vi "Performance Test.vi"() -> ()   [LabVIEW 2017]
uses:
  <vilib>/Simulation/Implementation/Shared/SIMSCR Execution Mode.ctl
  <vilib>/Simulation/Scripting/Companion Diagram/SimConfigNode/_simSolvers.ctl
  <vilib>/Simulation/Scripting/Companion Diagram/SimConfigNode/SimParams.ctl
  <vilib>/Simulation/Scripting/Companion Diagram/SimConfigNode/SimDog.xnode
  <vilib>/Simulation/Implementation/XNodeFramework/SimXNode/SimX.xnode
  FPGA_Read_Write.vi
  Manipulator/Inv Kin.vi
  Manipulator/Fwd Kin.vi
  Extras/type convert.vi
  <extravilib>/ChannelInstances/Tag-a[.](dbl).lvlib
  <extravilib>/ChannelInstances/Tag-bool.lvlib
  <vilib>/Platform/TimedLoop/XDataNode/wakeup.ctl
  <vilib>/Platform/TimedLoop/XDataNode/XDNodeRunTimeDep.lvlib
  <vilib>/Platform/TimedLoop/XDataNode/nitl_modes.ctl
  <vilib>/Platform/TimedLoop/XDataNode/timing_clust.ctl
  <vilib>/Platform/TimedLoop/XDataNode/XDataNode.xnode
  <extravilib>/ChannelInstances/Tag-c(bool,i32,str).lvlib
  <extravilib>/ChannelInstances/Tag-a[.](c(dbl,dbl)).lvlib
  Extras/NaN Check.vi
  <vilib>/rvi/interface/nirviReadWriteControl/nirviReadWriteControl.xnode
  <extravilib>/ChannelInstances/Tag-dbl.lvlib
  <vilib>/Analysis/baseanly.llb/Dot Product.vi
  <vilib>/Analysis/NI_AALBase.lvlib
  <vilib>/Analysis/baseanly.llb/Real Dot Product.vi
  <extravilib>/ChannelInstances/Tag-a[.](i32).lvlib
  Calibration/c PID.vi
  NiFpgaLv.dll
  <vilib>/Utility/error.llb/Error Cluster From Error Code.vi
  <vilib>/rvi/interface/Simulation/niFpgaSimulationCallBeginRW.vi
  <vilib>/rvi/errors/niLvFpgaAdjustHostInterfaceError.vi
  <vilib>/Simulation/Utility/Implementation/SIM Time.vi
  <vilib>/Simulation/Utility/Implementation/SIM Halt.vi
panel:
  out "Current Error":dbl
  out "Avg. Error":dbl
  out "Seconds per loop":dbl format="%#_3g"
  out "SM loop":i32=120971
  out "Number of loops \ncompleted":dbl=50.0
  in  "Error Threshold":dbl=0.2 format="%#_13g"
  out "Simulation Time":dbl=15.030000000000001
  out "Gains Motor 2":dbl[](array[numeric])=[60.0, 90.0, 2.0]
  out "Gains Motor 3":dbl[](array[numeric])=[60.0, 90.0, 2.0]
  out "Voltage Command 2":dbl[](array[numeric])=[0.4832188875674641, -1.217519090984242]
  in  "Integral 3":dbl(knob)=90.0 min=0.0 max=100.0 step=1.0 scale=0.0..100.0
  in  "Derivative 3":dbl(knob)=2.0 min=0.0 max=20.0 step=0.5 scale=0.0..10.0 scale format="%^#_6g"
  in  "Proportional 3":dbl(knob)=60.0 min=0.0 max=200.0 step=1.0 scale=0.0..200.0
  in  "Proportional 2":dbl(knob)=60.0 min=0.0 max=200.0 step=1.0 scale=0.0..200.0
  in  "Integral 2":dbl(knob)=90.0 min=0.0 max=100.0 step=1.0 scale=0.0..100.0
  in  "Derivative 2":dbl(knob)=2.0 min=0.0 max=20.0 step=0.5 scale=0.0..10.0 scale format="%^#_6g"
  out "End-effector\ntrajectory":cluster{dbl[], dbl[]}[](graph)
  out "Source Image":T1(plugin-control)
  in  "stop 3":bool
  out "Calibration":u32(slide) scale=1.0..3.0
  # "Proportional 0"
  # "Integral 0"
  # "Derivative 0"
  # "Proportional 1"
  # "Integral 1"
  # "Derivative 1"
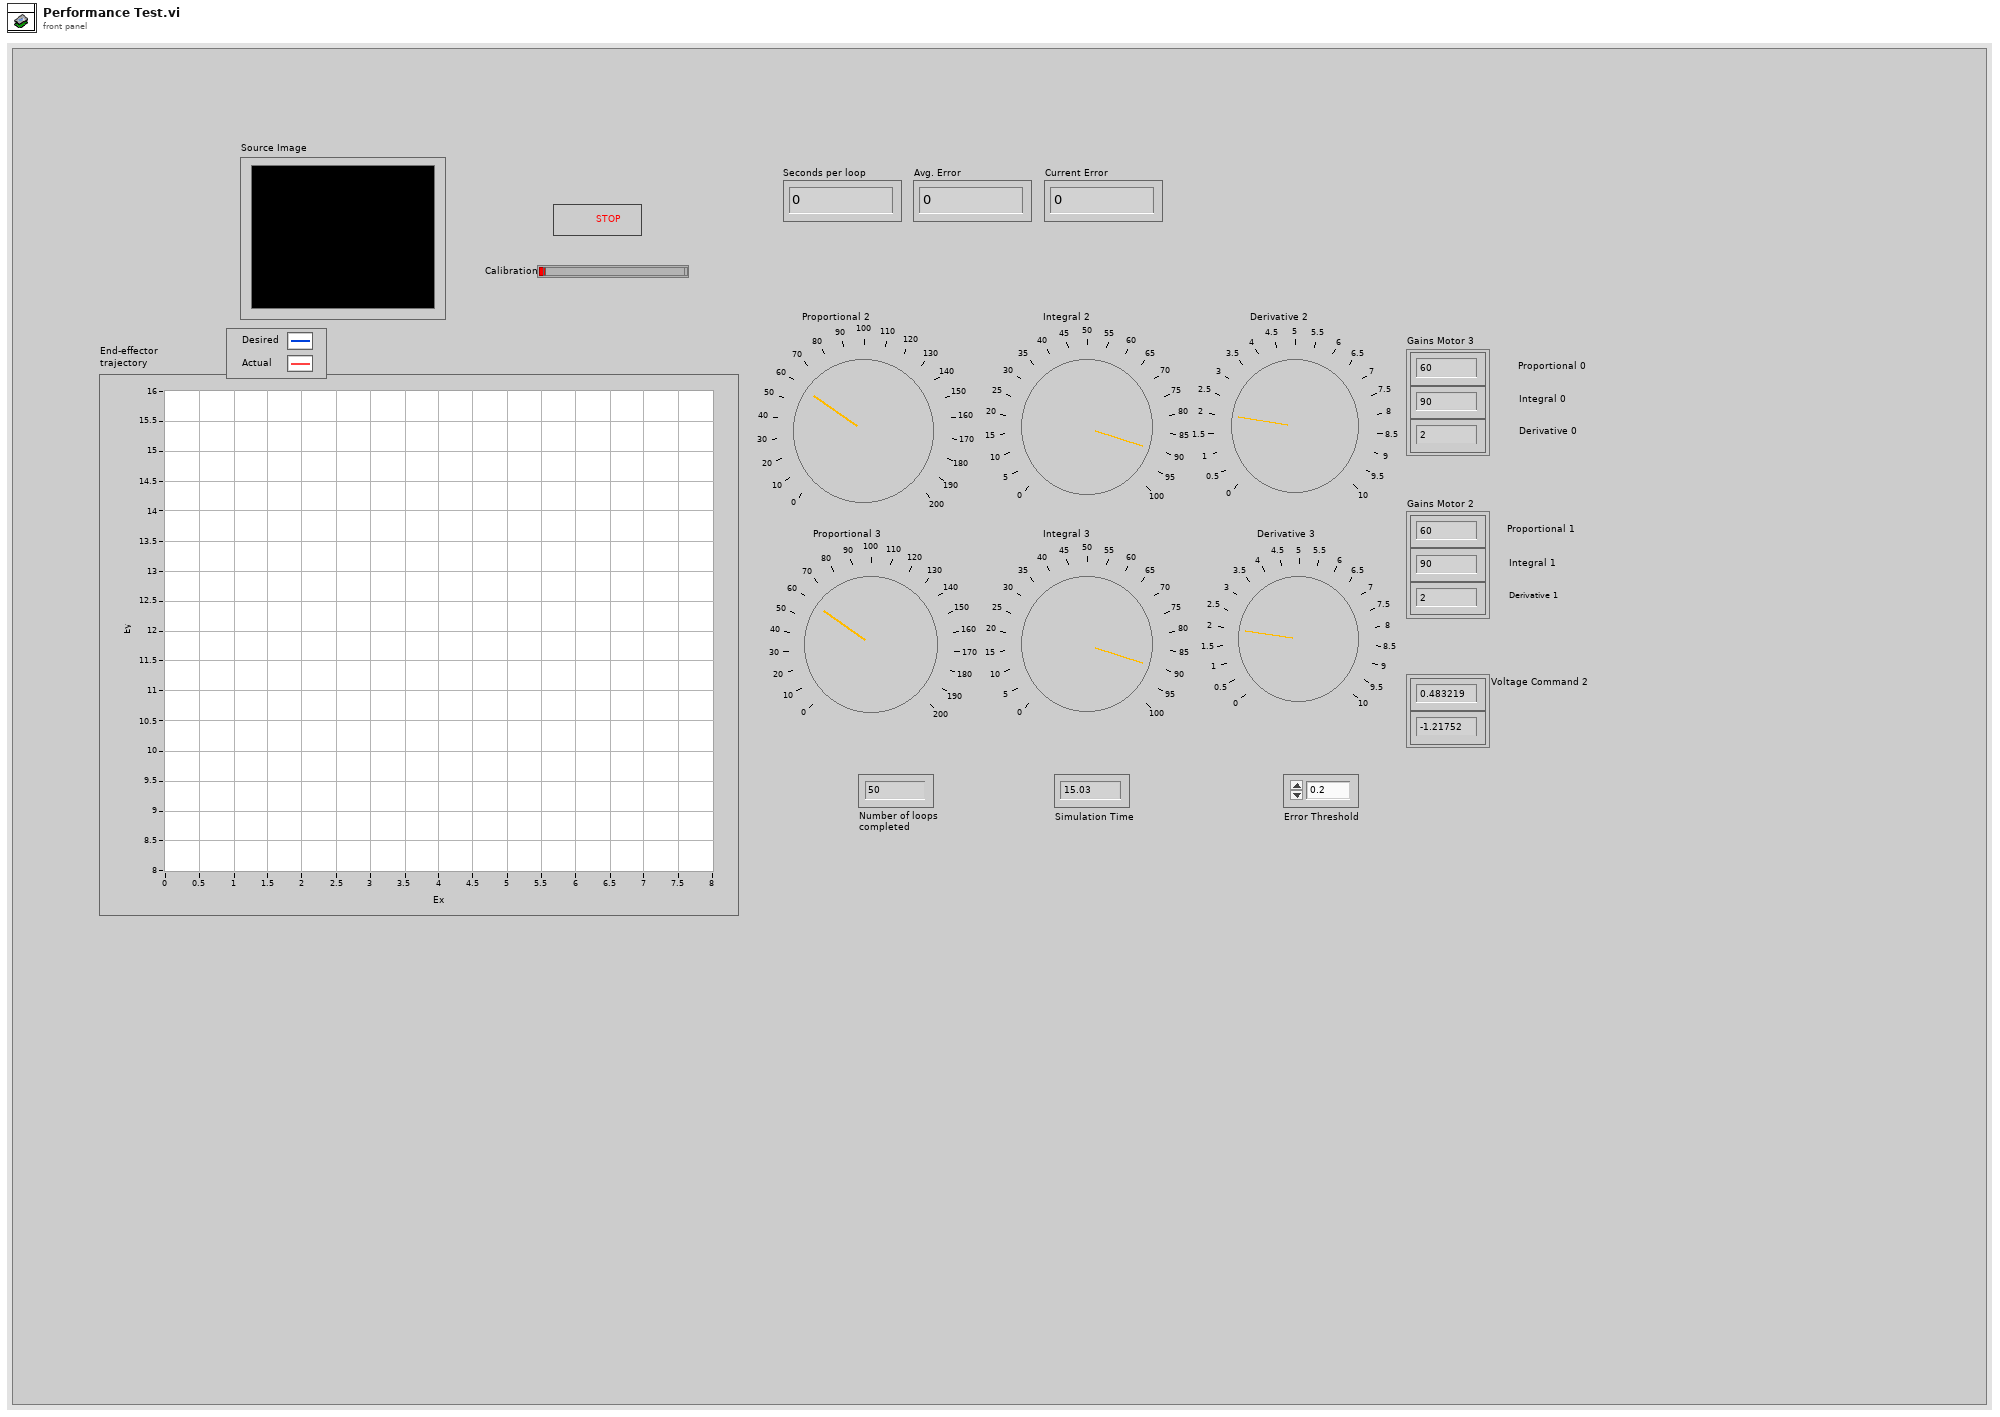
[diagram p1: front panel]
types:
  T1 = typedef "IMAQ Image.ctl" = refnum<image>
  T2 = typedef "QNET MS IO Cluster.ctl" = cluster{"Error":errorcluster, "Encoder Calibration Values":i32[], "Update Calibration":bool, "JPEG Resolutions":u16, "Raw Resolutions":u16, "Image Mode":enum16{"RAW RGB", "RAW Gray Scale", "JPEG"}, "FPGA Ref":refnum<k20>}
  T3 = typedef "XDNodeRunTimeDep.lvlib/timing_clust.ctl" = cluster{"Expected End [f-1]":u64, "Actual End [f-1]":u64, "Finished Late? [f-1]":bool, "Expected End [i-1]":u64, "Actual End [i-1]":u64, "Finished Late? [i-1]":bool, "Expected Start [i]":u64, "Actual Start [i]":u64, "Expected Start [f]":u64, "Actual Start [f]":u64, "Source Name":string, "Structure Name":string, "Period":i64, "Deadline":i64, "Offset":i64, "Start":i64, "Priority":i32, "Timeout":i32, "Mode":T4, "Wakeup Reason":T5, "Error":errorcluster, "Source Type":string, "Secondary Source Type":string, "Global End Time":u64, "Global Start Time":u64, "Frame Duration":u64, "Iteration Duration":u64, "Assigned CPU":i32, "I/O Scan Engine Mode":u32}
  T4 = typedef "XDNodeRunTimeDep.lvlib/nitl_modes.ctl" = enum32{"No Change", "Process missed periods, maintain original phase", "Discard missed periods, maintain original phase", "Process missed periods, ignore original phase", "Discard missed periods, ignore original phase"}
  T5 = typedef "XDNodeRunTimeDep.lvlib/wakeup.ctl" = enum32{"Normal", "Aborted", "Asynchronous wakeup", "Timing source error", "Timed loop error", "Timeout"}
  T6 = cluster{"Position":cluster{"x":sgl, "y":sgl}, "Angle":sgl, "Scale":sgl, "Score":sgl, "Bounding Box":cluster{"x":sgl, "y":sgl}[]}[]
  T7 = typedef "Tag-bool.lvlib/))Channel.ctl" = refnum<queue>
  T8 = typedef "Tag-c(bool,i32,str).lvlib/))Channel.ctl" = refnum<queue>
  T9 = typedef "Tag-a[.](i32).lvlib/))Channel.ctl" = refnum<queue>
  T10 = typedef "Tag-a[.](dbl).lvlib/))Channel.ctl" = refnum<queue>
  T11 = typedef "Tag-a[.](c(dbl,dbl)).lvlib/))Channel.ctl" = refnum<queue>
  T12 = typedef "Tag-dbl.lvlib/))Channel.ctl" = refnum<queue>
  T13 = cluster{"Numeric Control":dbl, "Numeric Control":dbl}[]
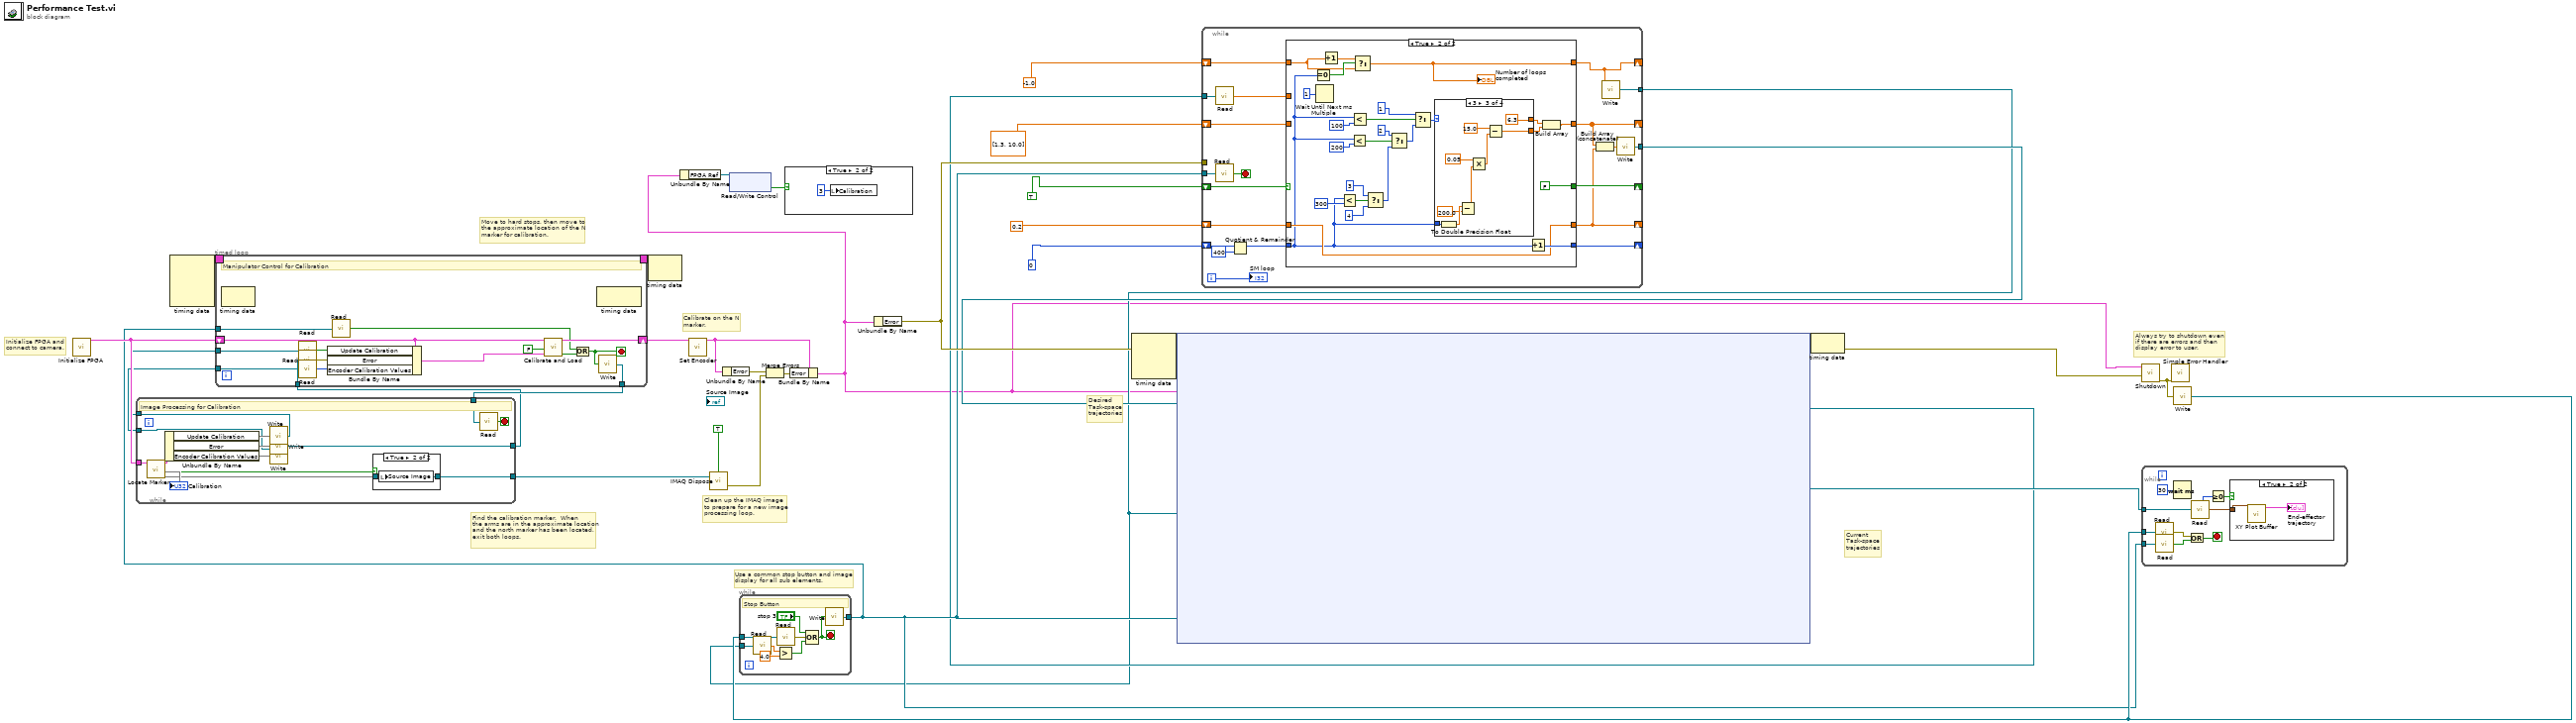
[diagram p0: block diagram]
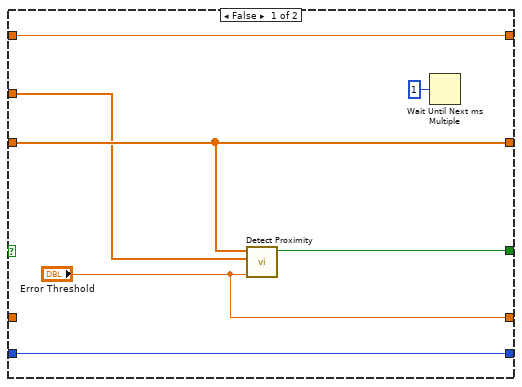
[diagram p2: hidden frame]
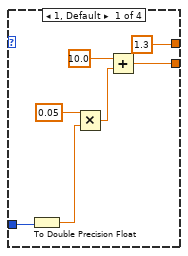
[diagram p3: hidden frame]
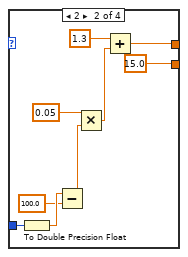
[diagram p4: hidden frame]
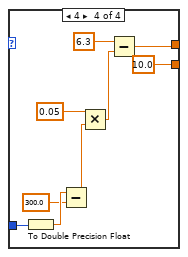
[diagram p5: hidden frame]
diagram:
  # "Current\nTask-space\ntrajectories"
  # "Desired\nTask-space\ntrajectories"
  # "Always try to shutdown even \nif there are errors and then \ndisplay error to user."
  # "Clean up the IMAQ image\nto prepare for a new image\nprocessing loop."
  # "Use a common stop button and image\ndisplay for all sub elements."
  # "Calibrate on the N\nmarker."
  # "Find the calibration marker.  When\nthe arms are in the approximate location\nand the north marker has been located,\nexit both loops."
  # "Move to hard stops, then move to\nthe approximate location of the N\nmarker for calibration."
  # "Initialize FPGA and\nconnect to camera."
  n1 = call "Initialize FPGA.vi"() -> ("IO Cluster Out"=w31:T2)  [unwired: 3 in]
  n2 = node-c288() -> (w33:T3)  [unwired: 4 in]
  n3 = while {
    tunnel: w31 -> [w44]
    tunnel: w30 -> [w47]
    tunnel: [w41] -> w27
    tunnel: [w36] -> w4
    tunnel: [w35] -> w3
    tunnel: [w34] -> w2
    stop <- w46 stop-if-true
    # "Image Processing for Calibration"
    n4 = call "Locate Marker.vi"("IO Cluster In"=w44) -> (0:w42, "New Image"=w43:bool, "Matches (pixel)"=w40:T6, 6:→"Calibration")  [unwired: 6 in, 1 out]
    n5 = Unbundle By Name(w40) -> ("Update Calibration"=w39, "Error"=w38, "Encoder Calibration Values"=w37)
    n6 = call <extravilib>:"Write.vi"("element"=w39) -> ("channel"=w36:T7)  [unwired: 1 out]
    n7 = call <extravilib>:"Write.vi"("element"=w38) -> ("channel"=w35:T8)  [unwired: 1 out]
    n8 = call <extravilib>:"Write.vi"("element"=w37) -> ("channel"=w34:T9)  [unwired: 1 out]
    n9 = case shown="True" w43 {
      tunnel: w42 -> [w48 w49]
      tunnel: [w48 w49] -> w41
      frame False {
      }
      frame True {
        n10 = local write "Source Image"(w49) -> ()
      }
    }
    n11 = call <extravilib>:"Read.vi"("channel"=w47) -> ("element"=w46:bool)  [unwired: 1 in, 1 out]
  }
  n12 = call "IMAQ Dispose"("All Images? (No)"=TRUE, "Image"=w27) -> ("error out"=w23:errorcluster)  [unwired: 4 in]
  n13 = timed-loop {
    shift-right: [w63] -> w29
    shift-left: w31 -> [w57]
    timing: w33 -> [_]
    timing-out: [_] -> w32
    tunnel: [w64] -> w30
    tunnel: w17 -> [w59]
    tunnel: w4 -> [w53]
    tunnel: w3 -> [w52]
    tunnel: w2 -> [w51]
    stop <- w61 stop-if-true
    # "Manipulator Control for Calibration"
    n14 = node-c288() -> ()  [unwired: 1 in, 1 out]
    n15 = call <extravilib>:"Read.vi"("channel"=w53) -> ("element"=w56:bool)  [unwired: 1 in, 1 out]
    n16 = call <extravilib>:"Read.vi"("channel"=w52) -> ("element"=w55:errorcluster)  [unwired: 1 in, 1 out]
    n17 = call <extravilib>:"Read.vi"("channel"=w51) -> ("element"=w54:i32[])  [unwired: 1 in, 1 out]
    n18 = Bundle By Name(cluster=w57, "Update Calibration"=w56, "Error"=w55, "Encoder Calibration Values"=w54) -> (w50:T2)
    n19 = call <extravilib>:"Read.vi"("channel"=w59) -> ("element"=w58:bool)  [unwired: 1 in, 1 out]
    n20 = call "Calibrate and Load.vi"(8:w50, "Always Calibrate"=FALSE, "IO Cluster In"=w57) -> ("Exit Loop"=w60:bool, "IO Cluster Out"=w63:T2)  [unwired: 6 in, 1 out]
    n21 = Or(x=w58, y=w60) -> (x .or. y?=w61:bool)
    n22 = node-c288() -> ()  [unwired: 1 in, 1 out]
    n23 = call <extravilib>:"Write.vi"("element"=w61) -> ("channel"=w64:T7)  [unwired: 1 out]
  }
  n24 = node-c288(w32) -> ()  [unwired: 1 out]
  n25 = call "Set Encoder.vi"("IO Cluster In"=w29) -> ("IO Cluster Out"=w26:T2)  [unwired: 10 in]
  n26 = Unbundle By Name(w26) -> ("Error"=w24:errorcluster)
  n27 = Merge Errors(w24, w23) -> (w25:errorcluster)
  n28 = Bundle By Name(cluster=w26, "Error"=w25) -> (w1:T2)
  n29 = Unbundle By Name(w1) -> ("FPGA Ref"=w16:refnum<k20>)
  n30 = xnode "Read/Write Control"("FPGA VI Reference In"=w16) -> ("Calibrated"=w15:bool)  [unwired: 1 in, 2 out]
  n31 = case shown="True" w15 {
    frame False {
    }
    frame True {
      n32 = local write "Calibration"(u32 3 ("Calibration")) -> ()
    }
  }
  n33 = Unbundle By Name(w1) -> ("Error"=w21:errorcluster)
  n34 = node-c288(w21) -> (w14:variant)  [unwired: 3 in]
  n35 = while {
    tunnel: [w76] -> w17
    tunnel: w18 -> [w75]
    tunnel: w5 -> [w71]
    stop <- w72 stop-if-true
    # "Stop Button"
    n36 = call <extravilib>:"Read.vi"("channel"=w71) -> ("element"=w70:dbl)  [unwired: 1 in, 1 out]
    n37 = Greater?(x=w70, y=4.0) -> (0:w68:bool)
    n38 = call <extravilib>:"Read.vi"("channel"=w75) -> ("element"=w74:errorcluster)  [unwired: 1 in, 1 out]
    n39 = Compound Arithmetic op=OR("stop 3", w74, w68) -> (w72:bool)
    n40 = call <extravilib>:"Write.vi"("element"=w72) -> ("channel"=w76:T7)  [unwired: 1 out]
  }
  n41 = node-c254 ("Control & Simulation Loop 3")(w14, w7, w17, w5, w1) -> (w13:variant, w6:T10, w19:T11)
  n42 = while {
    shift-right: [w94] -> _
    shift-left: TRUE -> [w96]
    shift-right: [w95] -> _
    shift-left: 0 -> [w93]
    tunnel: w21 -> [_]
    shift-right: [w84] -> _
    shift-left: 0.2 ("Threshold") -> [w89]
    shift-right: [w88] -> _
    shift-left: -1.0 -> [w87]
    shift-right: [w85] -> _
    shift-left: dbl[] [1.3, 10.0] -> [w86]
    tunnel: [w82] -> w7
    tunnel: w6 -> [w81]
    tunnel: w17 -> [w79]
    tunnel: [w77] -> w5
    i -> [w90]
    stop <- w78 stop-if-true
    n43 = call <extravilib>:"Read.vi"("channel"=w81) -> ("element"=w80:dbl[])  [unwired: 1 in, 1 out]
    n44 = call <extravilib>:"Read.vi"("channel"=w79) -> ("element"=w78:bool)  [unwired: 1 in, 1 out]
    n45 = Quotient & Remainder(x=w93, y=400) -> (x-y*floor(x/y)=w91:i32)  [unwired: 1 out]
    n46 = case shown="True" w96 {
      tunnel: w91 -> [w102 w111]
      tunnel: [w102 w113] -> w95
      tunnel: [w101 FALSE] -> w94
      tunnel: ["Error Threshold" w112] -> w84
      tunnel: w89 -> [_ w112]
      tunnel: [w100 w109] -> w88
      tunnel: w87 -> [w100 w107]
      tunnel: [w99 w104] -> w85
      tunnel: w86 -> [w99 _]
      tunnel: w80 -> [w98 _]
      frame False {
        n47 = call "Detect Proximity.vi"("Threshold"="Error Threshold", "E current"=w98, "E desired"=w99) -> ("Close Enough?"=w101:bool)  [unwired: 8 in]
        n48 = Wait Until Next ms Multiple(millisecond multiple=u32 1) -> ()  [unwired: 1 out]
      }
      frame True {
        n49 = Equal To 0?(x=w111) -> (x = 0?=w110:bool)
        n50 = Wait Until Next ms Multiple(millisecond multiple=u32 1) -> ()  [unwired: 1 out]
        n51 = Increment(x=w107) -> (x+1=w108:dbl)
        n52 = Less?(x=w111, y=300) -> (x < y?=w117:bool)
        n53 = Less?(x=w111, y=200) -> (x < y?=w122:bool)
        n54 = Less?(x=w111, y=100) -> (x < y?=w125:bool)
        n55 = Select(t=w108, s=w110, f=w107) -> (s? t:f=w109:dbl)
        "Number of loops \ncompleted" <- w109
        n56 = Select(t=3, s=w117, f=4 ("t")) -> (s? t:f=w118:i32)
        n57 = Select(t=2, s=w122, f=w118) -> (s? t:f=w119:i32)
        n58 = Select(t=1, s=w125, f=w119) -> (s? t:f=w114:i32)
        n59 = case shown="3" w114 {
          tunnel: w111 -> [w133 w141 w145 w156]
          tunnel: [1.3 w137 6.3 w155] -> w106
          tunnel: [w129 15.0 w146 10.0] -> w105
          frame 1, Default {
            n60 = To Double Precision Float(number=w133) -> (double precision float=w132:dbl)
            n61 = Multiply(x=0.05, y=w132) -> (x*y=w131:dbl)
            n62 = Add(x=10.0, y=w131) -> (x+y=w129:dbl)
          }
          frame 2 {
            n63 = To Double Precision Float(number=w141) -> (double precision float=w140:dbl)
            n64 = Subtract(x=w140, y=100.0) -> (x-y=w138:dbl)
            n65 = Multiply(x=0.05, y=w138) -> (x*y=w142:dbl)
            n66 = Add(x=1.3, y=w142) -> (x+y=w137:dbl)
          }
          frame 3 {
            n67 = To Double Precision Float(number=w145) -> (double precision float=w151:dbl)
            n68 = Subtract(x=w151, y=200.0) -> (x-y=w149:dbl)
            n69 = Multiply(x=0.05, y=w149) -> (x*y=w152:dbl)
            n70 = Subtract(x=15.0, y=w152) -> (x-y=w146:dbl)
          }
          frame 4 {
            n71 = To Double Precision Float(number=w156) -> (double precision float=w160:dbl)
            n72 = Subtract(x=w160, y=300.0) -> (x-y=w158:dbl)
            n73 = Multiply(x=0.05, y=w158) -> (x*y=w161:dbl)
            n74 = Subtract(x=6.3, y=w161) -> (x-y=w155:dbl)
          }
        }
        n75 = Increment(x=w111) -> (x+1=w113:i32)
        n76 = Build Array(w106, w105) -> (w104:dbl[])
      }
    }
    n77 = Build Array (concatenate)(w85, w84) -> (w83:dbl[])
    n78 = call <extravilib>:"Write.vi"("element"=w88) -> ("channel"=w77:T12)  [unwired: 1 out]
    n79 = call <extravilib>:"Write.vi"("element"=w83) -> ("channel"=w82:T10)  [unwired: 1 out]
    "SM loop" <- w90
  }
  n80 = node-c288(w13) -> (w20:errorcluster)
  n81 = call "Shutdown.vi"("Manipulator Loop"=w20, "IO Cluster In"=w1) -> ("Error"=w22:errorcluster)  [unwired: 9 in]
  n82 = call <vilib>:"Simple Error Handler.vi"("error in (no error)"=w22) -> ()  [unwired: 4 in, 5 out]
  n83 = call <extravilib>:"Write.vi"("element"=w22) -> ("channel"=w18:T8)  [unwired: 1 out]
  n84 = while {
    tunnel: w19 -> [w172]
    tunnel: w17 -> [w171]
    tunnel: w18 -> [w170]
    stop <- w169 stop-if-true
    n85 = call <extravilib>:"Read.vi"("channel"=w170) -> ("element"=w168:errorcluster)  [unwired: 1 in, 1 out]
    n86 = call <extravilib>:"Read.vi"("channel"=w171) -> ("element"=w167:bool)  [unwired: 1 in, 1 out]
    n87 = Wait (ms)(milliseconds to wait=u32 30) -> ()  [unwired: 1 out]
    n88 = Or(x=w168, y=w167) -> (x .or. y?=w169:bool)
    n89 = call <extravilib>:"Read.vi"("channel"=w172) -> ("missed"=w163:i32, "element"=w165:T13)  [unwired: 1 in]
    n90 = Greater Or Equal To 0?(x=w163) -> (x >= 0?=w164:bool)
    n91 = case shown="True" w164 {
      tunnel: w165 -> [_ w174]
      frame False {
      }
      frame True {
        n92 = call "XY Plot Buffer.vi"("Actual"=w174) -> ("Buffered Task Coordinates"=→"End-effector\ntrajectory":cluster{dbl[], dbl[]}[])  [unwired: 10 in]
      }
    }
  }
